vi "Grava_ArrayInFile_float.vi"(1 "format (%p)":string="%p", 2 "Array to save":sgl[](array[numeric]) format="%#_6p", 3 "file name":string, 4 "folder path":path) -> ()   [LabVIEW 2015, in "VIPM2.lvlib"]
doc: "Generic subVI to save an array into a text file, with format %08x.\nTo save: EQ_DATA+Report d'un Chip o Layer; GlobalReg; PixelReg."
uses:
  VIPM2.lvlib
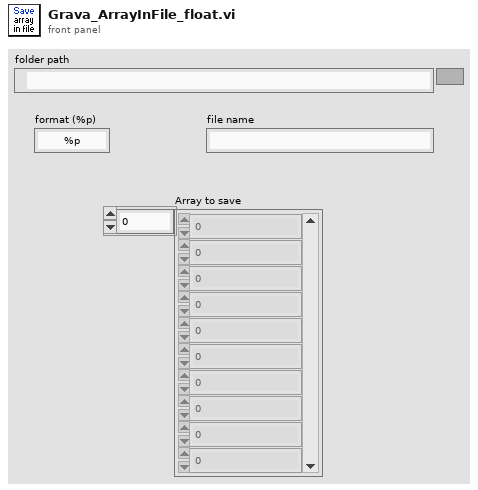
[diagram p1: front panel]
types:
  T1 = enum16{"open", "replace", "create", "open or create", "replace or create", "replace or create with confirmation"}
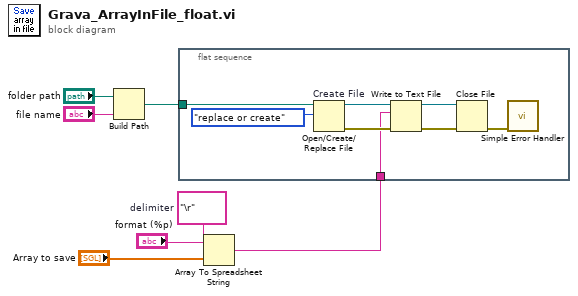
[diagram p0: block diagram]
diagram:
  w1 = "\r"  # delimiter
  n1 = Build Path(base path="folder path", name or relative path="file name") -> (appended path=w7:path)
  n2 = flat-sequence {
    tunnel: w7 -> [w15]
    tunnel: w3 -> [w8]
    frame #0 {
      n3 = Open/Create/Replace File "Create File"(file path (use dialog)=w15, operation (0:open)=T1."replace or create") -> (refnum out=w13:refnum<file>, error out=w12:errorcluster)  [unwired: 4 in, 1 out]
      n4 = Write to Text File(file (use dialog)=w13, text=w8, error in=w12) -> (refnum out=w11:refnum<file>, error out=w10:errorcluster)  [unwired: 1 in, 1 out]
      n5 = Close File(refnum=w11, error in=w10) -> (error out=w9:errorcluster)  [unwired: 1 out]
      n6 = call <vilib>:"Simple Error Handler.vi"("error in (no error)"=w9) -> ()  [unwired: 4 in, 5 out]
    }
  }
  n7 = Array To Spreadsheet String(delimiter (Tab)=w1, array="Array to save", 3:"format (%p)") -> (spreadsheet string=w3:string)
